vi "Untitled 3.vi"() -> ()   [LabVIEW 2011]
panel:
  out "0, 1":i16
  out "*(type *) &x 3":i32
  out "data string":string
  out "*(type *) &x 2":string
  out "*(type *) &x":string
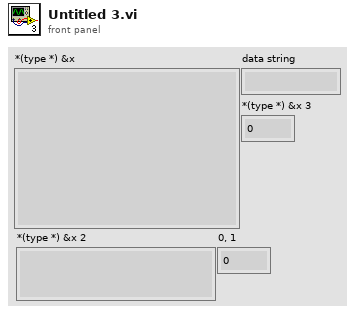
[diagram p1: front panel]
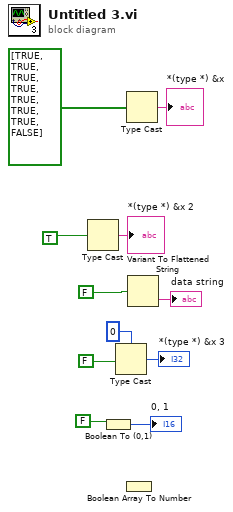
[diagram p0: block diagram]
diagram:
  n1 = Type Cast(x=TRUE) -> (*(type *) &x=→"*(type *) &x 2":string)  [unwired: 1 in]
  n2 = Boolean To (0,1)(Boolean=FALSE) -> (0, 1=→"0, 1":i16)
  n3 = Type Cast(type=0, x=FALSE) -> (*(type *) &x=→"*(type *) &x 3":i32)
  n4 = Boolean Array To Number() -> ()  [unwired: 1 in, 1 out]
  n5 = Type Cast(x=bool[] [TRUE, TRUE, TRUE, TRUE, TRUE, TRUE, TRUE, FALSE]) -> (*(type *) &x=→"*(type *) &x":string)  [unwired: 1 in]
  n6 = Variant To Flattened String(Variant=FALSE) -> (data string=→"data string":string)  [unwired: 1 out]
